vi "Get COM Descriptor from VISA.vi"(7 "To ASCII? (True)":bool=TRUE, 8 "error in (no error)":errorcluster, 10 "Generate error if no COM port found? (False)":bool, 11 "VISA resource name":refnum<visa-resource-name>) -> (0 "error out":errorcluster, 1 "COM port Descriptor":string, 2 "COM port":T1, 3 "VISA out":refnum<visa-resource-name>)   [LabVIEW 2020, in "Get COM Descriptor.lvlib"]
doc: "Get COM port descriptor string from VISA resource. Option To ASCII? will try to remove utf8 symbols (replaces accents with basic alphabet).\n\nDetails: https://github.com/smaslan/get-com-descriptor"
uses:
  Get COM Descriptor.lvlib
  COM port.ctl
  <vilib>/regexp/Match Regular Expression.xnode
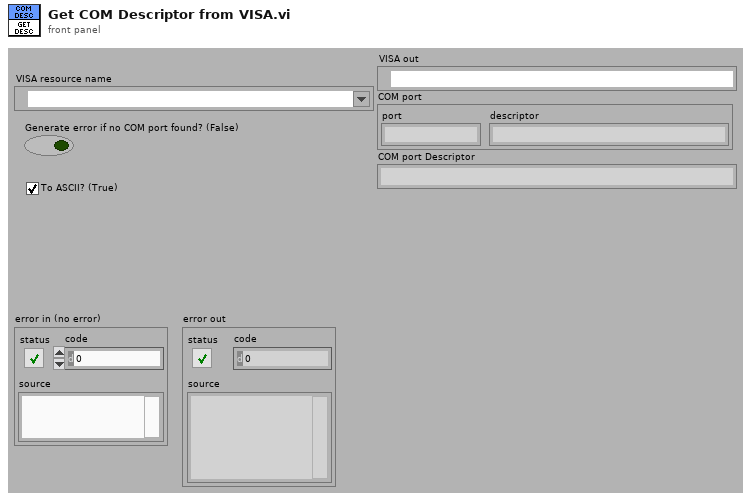
[diagram p1: front panel]
types:
  T1 = typedef "Get COM Descriptor.lvlib/COM port.ctl" = cluster{"port":string, "descriptor":string}
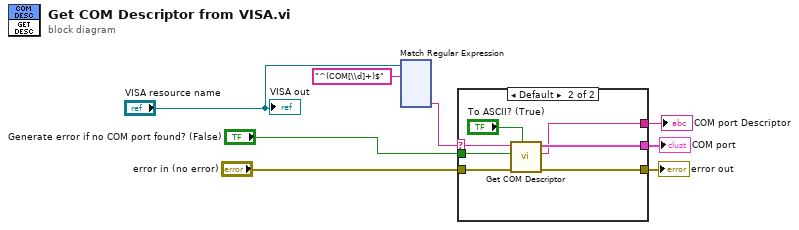
[diagram p0: block diagram]
diagram:
  n1 = xnode "Match Regular Expression"("input string"="VISA resource name", "regular expression"="^(COM[\\d]+)$") -> ("submatch 1"=w3:string)  [unwired: 4 in, 5 out]
  n2 = case shown="Default" w3 {
    selector: w3 -> [_ w13]
    tunnel: "error in (no error)" -> [w9 w16]
    tunnel: [w9 w15] -> w5
    tunnel: "Generate error if no COM port found? (False)" -> [_ w14]
    tunnel: [_ w12] -> w2
    tunnel: [_ w11] -> w1
    frame "" {
    }
    frame Default {
      n3 = call "Get COM Descriptor.vi"("To ASCII? (True)"="To ASCII? (True)", "error in (no error)"=w16, "Generate error if no COM port found? (False)"=w14, "COM name"=w13) -> ("error out"=w15:errorcluster, "COM port Descriptor"=w11:string, "COM port"=w12:T1)  [unwired: 5 in]
    }
  }
  "error out" <- w5
  "COM port" <- w2
  "COM port Descriptor" <- w1
  "VISA out" <- "VISA resource name"
